vi "Get User Palette Choice.vi"(8 "Error In":errorcluster, 9 "Inverse (F)":bool, 10 "Interpolated Color Scale Definition":T1, 11 "Palette":string) -> (0 "Error Out":errorcluster, 1 "Palette Colors":u32[](array[numeric]), 2 "Palette Type":T2 items=["Grayscale", "Binary", "Gradient", "Rainbow", "Temperature", "User Defined", "Binary 16 Bit", "Gradient 16 Bit", "Rainbow 16 Bit", "Temperature 16 Bit", "User Defined 16 Bit"], 3 "Palette Name (# Colors)":string, 4 "Palette set?":bool, 5 "Brewer Palette?":bool, 6 "Interpolate?":bool)   [LabVIEW 2021]
uses:
  Image/Image Display Palette Type.ctl
  Interpolated Color Scale Definition.ctl
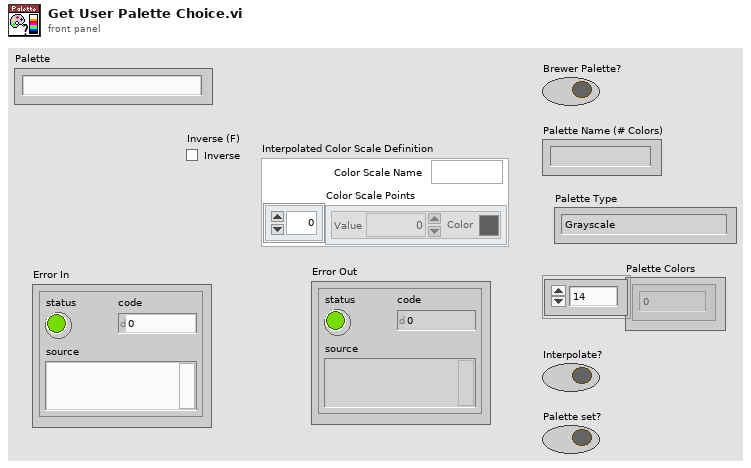
[diagram p1: front panel]
types:
  T1 = typedef "Interpolated Color Scale Definition.ctl" = cluster{"Color Scale Points":cluster{"Value":dbl, "Color":u32}[], "Color Scale Name":string}
  T2 = typedef "Image Display Palette Type.ctl" = u32
  T3 = typedef "Color Brewer Palette.ctl" = cluster{"Color Array":u32[], "Palette Name":string, "Number of Colors":i32, "Palette Category":string, "Color Blind Safe":bool, "Printer Friendly":bool, "Photocopy Safe":bool}
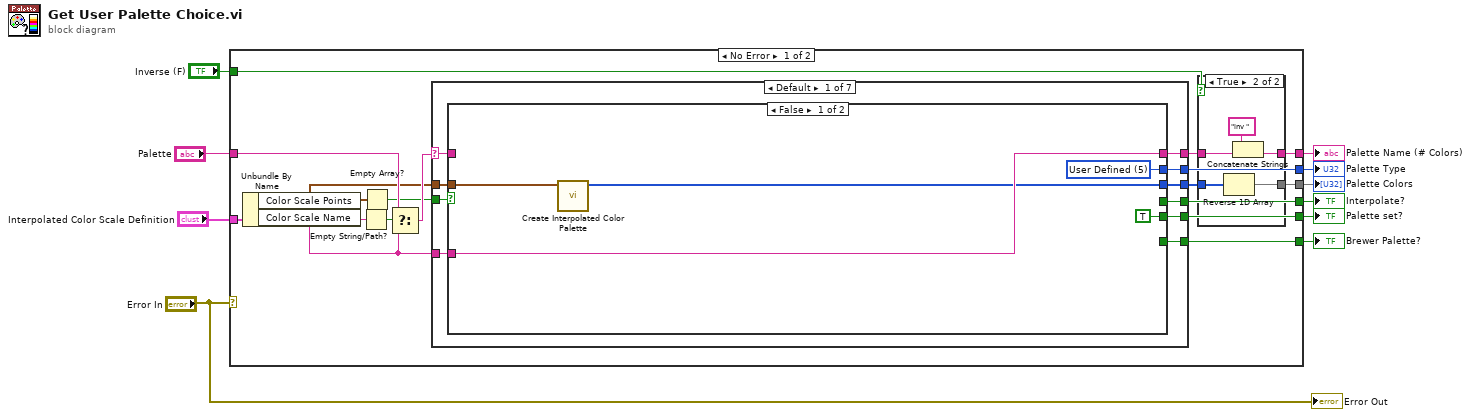
[diagram p0: block diagram]
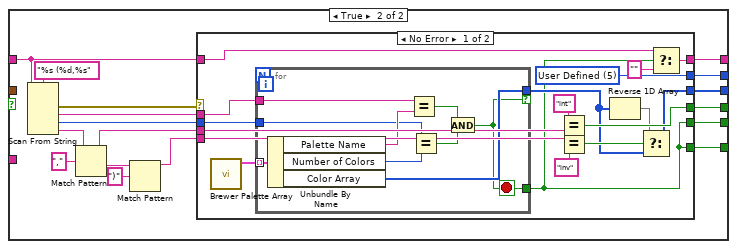
[diagram p3: hidden frame]
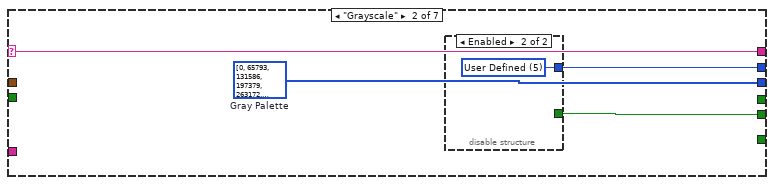
[diagram p5: hidden frame]
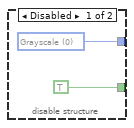
[diagram p6: hidden frame]
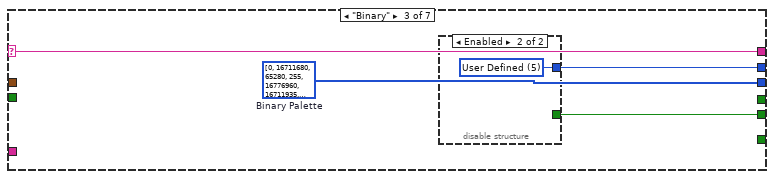
[diagram p7: hidden frame]
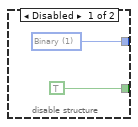
[diagram p8: hidden frame]
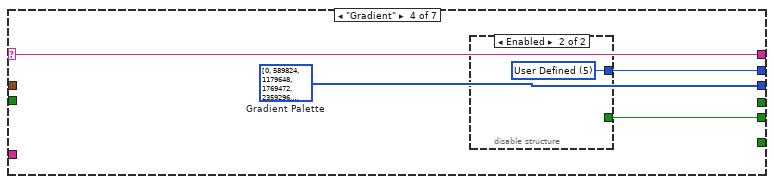
[diagram p9: hidden frame]
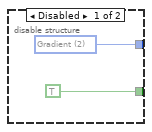
[diagram p10: hidden frame]
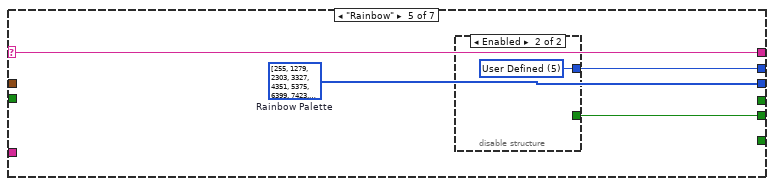
[diagram p11: hidden frame]
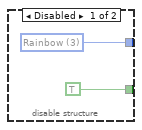
[diagram p12: hidden frame]
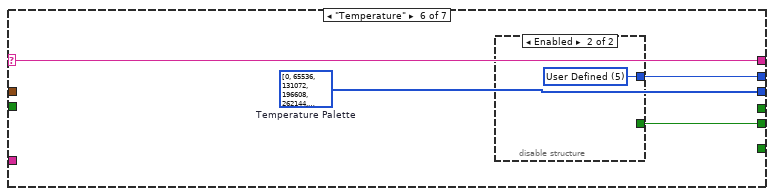
[diagram p13: hidden frame]
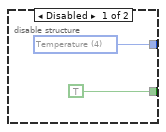
[diagram p14: hidden frame]
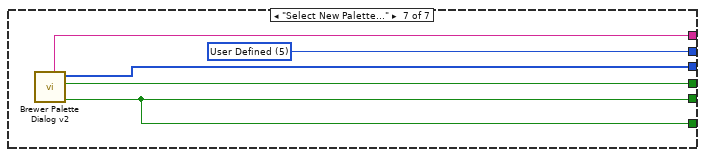
[diagram p15: hidden frame]
diagram:
  n1 = case shown="No Error" "Error In" {
    tunnel: [w20 _] -> w10
    tunnel: [w26 _] -> w9
    tunnel: [w18 _] -> w8
    tunnel: [w25 _] -> w7
    tunnel: [w24 _] -> w6
    tunnel: [w23 _] -> w5
    tunnel: "Palette" -> [w14 _]
    tunnel: "Inverse (F)" -> [w22 _]
    tunnel: "Interpolated Color Scale Definition" -> [w17 _]
    frame No Error {
      n2 = Unbundle By Name(w17) -> ("Color Scale Points"=w11:cluster{"Value":dbl, "Color":u32}[], "Color Scale Name"=w12:string)
      n3 = Empty String/Path?(string/path=w12) -> (empty?=w16:bool)
      n4 = Empty Array?(array=w11) -> (empty?=w13:bool)
      n5 = Select(t=w14, s=w16, f=w12) -> (s? t:f=w15:string)
      n6 = case shown="Default" w15 {
        selector: w15 -> [w37 w94 w101 w108 w115 w122 _]
        tunnel: [w41 w92 w99 w106 w113 w120 w131] -> w23
        tunnel: [w39 w95 w102 w109 w116 w123 w130] -> w24
        tunnel: [w42 _ _ _ _ _ w130] -> w25
        tunnel: [w43 w93 w100 w107 w114 w121 w129] -> w19
        tunnel: [w38 _ _ _ _ _ w128] -> w26
        tunnel: [w40 w94 w101 w108 w115 w122 w127] -> w21
        tunnel: w13 -> [w36 _ _ _ _ _ _]
        tunnel: w12 -> [w35 _ _ _ _ _ _]
        tunnel: w11 -> [w34 _ _ _ _ _ _]
        frame Default {
          n7 = case shown="False" w36 {
            tunnel: [w45 w62] -> w43
            tunnel: [_ w61] -> w42
            tunnel: [w47 w60] -> w41
            tunnel: [w48 w59] -> w40
            tunnel: [TRUE w58] -> w39
            tunnel: [_ w57] -> w38
            tunnel: w37 -> [_ w54]
            tunnel: w35 -> [w48 _]
            tunnel: w34 -> [w46 _]
            frame False {
              w47 = T2 5 items=["Grayscale", "Binary", "Gradient", "Rainbow", "Temperature", "User Defined", "Binary 16 Bit", "Gradient 16 Bit", "Rainbow 16 Bit", "Temperature 16 Bit", "User Defined 16 Bit"] ("Palette:Palette Type")
              n8 = call "Create Interpolated Color Palette.vi"("Color Scale Points"=w46) -> ("Interpolated Color Scale"=w45:u32[])  [unwired: 9 in, 1 out]
            }
            frame True {
              n9 = Scan From String(format string="%s (%d,%s", input string=w54) -> (error out=w65:errorcluster, output 1=w63:string, output 2=w64:i32, output 3=w52:string)  [unwired: 5 in, 2 out]
              n10 = Match Pattern(string=w52, regular expression=",") -> (before substring=w56:string, after substring=w50:string)  [unwired: 1 in, 2 out]
              n11 = Match Pattern(string=w50, regular expression=")") -> (before substring=w55:string)  [unwired: 1 in, 3 out]
              n12 = case shown="No Error" w65 {
                tunnel: w64 -> [w80 _]
                tunnel: w63 -> [w81 _]
                tunnel: [w70 _] -> w62
                tunnel: [w68 _] -> w61
                tunnel: [w79 _] -> w60
                tunnel: [w66 _] -> w59
                tunnel: [w68 _] -> w58
                tunnel: w56 -> [w78 _]
                tunnel: w55 -> [w75 _]
                tunnel: [w76 _] -> w57
                tunnel: w54 -> [w69 _]
                frame No Error {
                  w79 = T2 5 items=["Grayscale", "Binary", "Gradient", "Rainbow", "Temperature", "User Defined", "Binary 16 Bit", "Gradient 16 Bit", "Rainbow 16 Bit", "Temperature 16 Bit", "User Defined 16 Bit"] ("Palette:Palette Type")
                  n13 = call "Brewer Palette Array.vi"() -> ("Color Brewer Palette Array"=w82:T3[])  [unwired: 9 in]
                  n14 = for {
                    tunnel: w82 -> [w91] mode=indexing
                    tunnel: w81 -> [w84]
                    tunnel: w80 -> [w88]
                    tunnel: [w85] -> w72 if=w83
                    tunnel: [w83] -> w68
                    stop <- w83 stop-if-true
                    n15 = Unbundle By Name(w91) -> ("Palette Name"=w90:string, "Number of Colors"=w89:i32, "Color Array"=w85:u32[])
                    n16 = Equal?(x=w84, y=w90) -> (x = y?=w87:bool)
                    n17 = Equal?(x=w88, y=w89) -> (x = y?=w86:bool)
                    n18 = And(x=w87, y=w86) -> (x .and. y?=w83:bool)
                  }
                  n19 = Equal?(x="int", y=w78) -> (x = y?=w76:bool)
                  n20 = Equal?(x=w75, y="inv" ("x")) -> (x = y?=w73:bool)
                  n21 = Reverse 1D Array(array=w72) -> (reversed array=w71:u32[])
                  n22 = Select(t=w71, s=w73, f=w72) -> (s? t:f=w70:u32[])
                  n23 = Select(t=w69, s=w68, f="") -> (s? t:f=w66:string)
                }
                frame Error {
                }
              }
            }
          }
        }
        frame "Grayscale" {
          w93 = u32[] [0, 65793, 131586, 197379, 263172, 328965, 394758, 460551, 526344, 592137, 657930, 723723, 789516, 855309, 921102, 986895, 1052688, 1118481, 1184274, 1250067, 1315860, 1381653, 1447446, 1513239, 1579032, 1644825, 1710618, 1776411, 1842204, 1907997, 1973790, 2039583, 2105376, 2171169, 2236962, 2302755, 2368548, 2434341, 2500134, 2565927, 2631720, 2697513, 2763306, 2829099, 2894892, 2960685, 3026478, 3092271, 3158064, 3223857, 3289650, 3355443, 3421236, 3487029, 3552822, 3618615, 3684408, 3750201, 3815994, 3881787, 3947580, 4013373, 4079166, 4144959, 4210752, 4276545, 4342338, 4408131, 4473924, 4539717, 4605510, 4671303, 4737096, 4802889, 4868682, 4934475, 5000268, 5066061, 5131854, 5197647, 5263440, 5329233, 5395026, 5460819, 5526612, 5592405, 5658198, 5723991, 5789784, 5855577, 5921370, 5987163, 6052956, 6118749, 6184542, 6250335, 6316128, 6381921, 6447714, 6513507, 6579300, 6645093, 6710886, 6776679, 6842472, 6908265, 6974058, 7039851, 7105644, 7171437, 7237230, 7303023, 7368816, 7434609, 7500402, 7566195, 7631988, 7697781, 7763574, 7829367, 7895160, 7960953, 8026746, 8092539, 8158332, 8224125, 8289918, 8355711, 8421504, 8487297, 8553090, 8618883, 8684676, 8750469, 8816262, 8882055, 8947848, 9013641, 9079434, 9145227, 9211020, 9276813, 9342606, 9408399, 9474192, 9539985, 9605778, 9671571, 9737364, 9803157, 9868950, 9934743, 10000536, 10066329, 10132122, 10197915, 10263708, 10329501, 10395294, 10461087, 10526880, 10592673, 10658466, 10724259, 10790052, 10855845, 10921638, 10987431, 11053224, 11119017, 11184810, 11250603, 11316396, 11382189, 11447982, 11513775, 11579568, 11645361, 11711154, 11776947, 11842740, 11908533, 11974326, 12040119, 12105912, 12171705, 12237498, 12303291, 12369084, 12434877, 12500670, 12566463, 12632256, 12698049, 12763842, 12829635, 12895428, 12961221, 13027014, 13092807, 13158600, 13224393, 13290186, 13355979, 13421772, 13487565, 13553358, 13619151, 13684944, 13750737, 13816530, 13882323, 13948116, 14013909, 14079702, 14145495, 14211288, 14277081, 14342874, 14408667, 14474460, 14540253, 14606046, 14671839, 14737632, 14803425, 14869218, 14935011, 15000804, 15066597, 15132390, 15198183, 15263976, 15329769, 15395562, 15461355, 15527148, 15592941, 15658734, 15724527, 15790320, 15856113, 15921906, 15987699, 16053492, 16119285, 16185078, 16250871, 16316664, 16382457, 16448250, 16514043, 16579836, 16645629, 16711422, 16777215]  # Gray Palette
          n24 = disable-structure shown="Enabled" {
            disable-tunnel: [TRUE _] -> w95
            disable-tunnel: [w96 w98] -> w92
            frame Disabled {
              w96 = T2 0 items=["Grayscale", "Binary", "Gradient", "Rainbow", "Temperature", "User Defined", "Binary 16 Bit", "Gradient 16 Bit", "Rainbow 16 Bit", "Temperature 16 Bit", "User Defined 16 Bit"] ("Palette:Palette Type")
            }
            frame Enabled {
              w98 = T2 5 items=["Grayscale", "Binary", "Gradient", "Rainbow", "Temperature", "User Defined", "Binary 16 Bit", "Gradient 16 Bit", "Rainbow 16 Bit", "Temperature 16 Bit", "User Defined 16 Bit"] ("Palette:Palette Type")
            }
          }
        }
        frame "Binary" {
          w100 = u32[] [0, 16711680, 65280, 255, 16776960, 16711935, 65535, 16744192, 16711807, 8388352, 8323327, 32767, 65407, 16744319, 8388479, 8355839, 16711680, 65280, 255, 16776960, 16711935, 65535, 16744192, 16711807, 8388352, 8323327, 32767, 65407, 16744319, 8388479, 8355839, 16711680, 65280, 255, 16776960, 16711935, 65535, 16744192, 16711807, 8388352, 8323327, 32767, 65407, 16744319, 8388479, 8355839, 16711680, 65280, 255, 16776960, 16711935, 65535, 16744192, 16711807, 8388352, 8323327, 32767, 65407, 16744319, 8388479, 8355839, 16711680, 65280, 255, 16776960, 16711935, 65535, 16744192, 16711807, 8388352, 8323327, 32767, 65407, 16744319, 8388479, 8355839, 16711680, 65280, 255, 16776960, 16711935, 65535, 16744192, 16711807, 8388352, 8323327, 32767, 65407, 16744319, 8388479, 8355839, 16711680, 65280, 255, 16776960, 16711935, 65535, 16744192, 16711807, 8388352, 8323327, 32767, 65407, 16744319, 8388479, 8355839, 16711680, 65280, 255, 16776960, 16711935, 65535, 16744192, 16711807, 8388352, 8323327, 32767, 65407, 16744319, 8388479, 8355839, 16711680, 65280, 255, 16776960, 16711935, 65535, 16744192, 16711807, 8388352, 8323327, 32767, 65407, 16744319, 8388479, 8355839, 16711680, 65280, 255, 16776960, 16711935, 65535, 16744192, 16711807, 8388352, 8323327, 32767, 65407, 16744319, 8388479, 8355839, 16711680, 65280, 255, 16776960, 16711935, 65535, 16744192, 16711807, 8388352, 8323327, 32767, 65407, 16744319, 8388479, 8355839, 16711680, 65280, 255, 16776960, 16711935, 65535, 16744192, 16711807, 8388352, 8323327, 32767, 65407, 16744319, 8388479, 8355839, 16711680, 65280, 255, 16776960, 16711935, 65535, 16744192, 16711807, 8388352, 8323327, 32767, 65407, 16744319, 8388479, 8355839, 16711680, 65280, 255, 16776960, 16711935, 65535, 16744192, 16711807, 8388352, 8323327, 32767, 65407, 16744319, 8388479, 8355839, 16711680, 65280, 255, 16776960, 16711935, 65535, 16744192, 16711807, 8388352, 8323327, 32767, 65407, 16744319, 8388479, 8355839, 16711680, 65280, 255, 16776960, 16711935, 65535, 16744192, 16711807, 8388352, 8323327, 32767, 65407, 16744319, 8388479, 8355839, 16711680, 65280, 255, 16776960, 16711935, 65535, 16744192, 16711807, 8388352, 8323327, 32767, 65407, 16744319, 8388479, 16777215]  # Binary Palette
          n25 = disable-structure shown="Enabled" {
            disable-tunnel: [TRUE _] -> w102
            disable-tunnel: [w103 w105] -> w99
            frame Disabled {
              w103 = T2 1 items=["Grayscale", "Binary", "Gradient", "Rainbow", "Temperature", "User Defined", "Binary 16 Bit", "Gradient 16 Bit", "Rainbow 16 Bit", "Temperature 16 Bit", "User Defined 16 Bit"] ("Palette:Palette Type")
            }
            frame Enabled {
              w105 = T2 5 items=["Grayscale", "Binary", "Gradient", "Rainbow", "Temperature", "User Defined", "Binary 16 Bit", "Gradient 16 Bit", "Rainbow 16 Bit", "Temperature 16 Bit", "User Defined 16 Bit"] ("Palette:Palette Type")
            }
          }
        }
        frame "Gradient" {
          w107 = u32[] [0, 589824, 1179648, 1769472, 2359296, 2949120, 3538944, 4128768, 4718592, 5308416, 5898240, 6488064, 7077888, 7667712, 8257536, 8847360, 9437184, 9699328, 9961472, 10223616, 10485760, 10747904, 11010048, 11272192, 11534336, 11796480, 12058624, 12320768, 12582912, 12845056, 13107200, 13369344, 13631488, 13762560, 13893632, 14024704, 14155776, 14286848, 14417920, 14548992, 14680064, 14811136, 14942208, 15073280, 15204352, 15335424, 15466496, 15597568, 15728640, 15730176, 15731712, 15733248, 15734784, 15736320, 15737856, 15739392, 15740928, 15742464, 15744000, 15745536, 15747072, 15748608, 15750144, 15751680, 15753216, 15754240, 15755264, 15756288, 15757312, 15758336, 15759360, 15760384, 15761408, 15762432, 15763456, 15764480, 15765504, 15766528, 15767552, 15768576, 15769600, 15704832, 15640064, 15575296, 15510528, 15445760, 15380992, 15316224, 15251456, 15186688, 15121920, 15057152, 14992384, 14927616, 14862848, 14798080, 14733312, 14471680, 14210048, 13948416, 13686784, 13425152, 13163520, 12901888, 12640256, 12378624, 12116992, 11855360, 11593728, 11332096, 11070464, 10808832, 10547200, 10416134, 10285068, 10154002, 10022936, 9891870, 9760804, 9629738, 9498672, 9367606, 9236540, 9105474, 8974408, 8843342, 8712276, 8581210, 8450144, 8384613, 8319082, 8253551, 8188020, 8122489, 8056958, 7991427, 7925896, 7860365, 7794834, 7729303, 7663772, 7598241, 7532710, 7467179, 7401648, 7335603, 7269558, 7203513, 7137468, 7071423, 7005378, 6939333, 6873288, 6807243, 6741198, 6675153, 6609108, 6543063, 6477018, 6410973, 6344928, 6410465, 6476002, 6541539, 6607076, 6672613, 6738150, 6803687, 6869224, 6934761, 7000298, 7065835, 7131372, 7196909, 7262446, 7327983, 7393520, 7459312, 7525104, 7590896, 7656688, 7722480, 7788272, 7854064, 7919856, 7985648, 8051440, 8117232, 8183024, 8248816, 8314608, 8380400, 8446192, 8577519, 8708846, 8840173, 8971500, 9102827, 9234154, 9365481, 9496808, 9628135, 9759462, 9890789, 10022116, 10153443, 10284770, 10416097, 10547424, 10678496, 10809568, 10940640, 11071712, 11202784, 11333856, 11464928, 11596000, 11727072, 11858144, 11989216, 12120288, 12251360, 12382432, 12513504, 12644576, 12775648, 12906720, 13037792, 13168864, 13299936, 13431008, 13562080, 13693152, 13824224, 13955296, 14086368, 14217440, 14348512, 14479584, 14610656, 14741728, 14807265, 14872802, 14938339, 15003876, 15069413, 15134950, 15200487, 15266024, 15331561, 15397098, 15462635, 15528172, 15593709, 15659246, 15724783]  # Gradient Palette
          n26 = disable-structure shown="Enabled" {
            disable-tunnel: [TRUE _] -> w109
            disable-tunnel: [w110 w112] -> w106
            frame Disabled {
              w110 = T2 2 items=["Grayscale", "Binary", "Gradient", "Rainbow", "Temperature", "User Defined", "Binary 16 Bit", "Gradient 16 Bit", "Rainbow 16 Bit", "Temperature 16 Bit", "User Defined 16 Bit"] ("Palette:Palette Type")
            }
            frame Enabled {
              w112 = T2 5 items=["Grayscale", "Binary", "Gradient", "Rainbow", "Temperature", "User Defined", "Binary 16 Bit", "Gradient 16 Bit", "Rainbow 16 Bit", "Temperature 16 Bit", "User Defined 16 Bit"] ("Palette:Palette Type")
            }
          }
        }
        frame "Rainbow" {
          w114 = u32[] [255, 1279, 2303, 3327, 4351, 5375, 6399, 7423, 8447, 9471, 10495, 11519, 12543, 13567, 14591, 15615, 16639, 17663, 18687, 19711, 20735, 21759, 22783, 23807, 24831, 25855, 26879, 27903, 28927, 29951, 30975, 31999, 33023, 34047, 35071, 36095, 37119, 38143, 39167, 40191, 41215, 42239, 43263, 44287, 45311, 46335, 47359, 48383, 49407, 50431, 51455, 52479, 53503, 54527, 55551, 56575, 57599, 58623, 59647, 60671, 61695, 62719, 63743, 64767, 65535, 65531, 65527, 65523, 65519, 65515, 65511, 65507, 65503, 65499, 65495, 65491, 65487, 65483, 65479, 65475, 65471, 65467, 65463, 65459, 65455, 65451, 65447, 65443, 65439, 65435, 65431, 65427, 65423, 65419, 65415, 65411, 65407, 65403, 65399, 65395, 65391, 65387, 65383, 65379, 65375, 65371, 65367, 65363, 65359, 65355, 65351, 65347, 65343, 65339, 65335, 65331, 65327, 65323, 65319, 65315, 65311, 65307, 65303, 65299, 65295, 65291, 65287, 65283, 65280, 327424, 589568, 851712, 1113856, 1376000, 1638144, 1900288, 2162432, 2424576, 2686720, 2948864, 3211008, 3473152, 3735296, 3997440, 4259584, 4521728, 4783872, 5046016, 5308160, 5570304, 5832448, 6094592, 6356736, 6618880, 6881024, 7143168, 7405312, 7667456, 7929600, 8191744, 8453888, 8716032, 8978176, 9240320, 9502464, 9764608, 10026752, 10288896, 10551040, 10813184, 11075328, 11337472, 11599616, 11861760, 12123904, 12386048, 12648192, 12910336, 13172480, 13434624, 13696768, 13958912, 14221056, 14483200, 14745344, 15007488, 15269632, 15531776, 15793920, 16056064, 16318208, 16580352, 16776960, 16775936, 16774912, 16773888, 16772864, 16771840, 16770816, 16769792, 16768768, 16767744, 16766720, 16765696, 16764672, 16763648, 16762624, 16761600, 16760576, 16759552, 16758528, 16757504, 16756480, 16755456, 16754432, 16753408, 16752384, 16751360, 16750336, 16749312, 16748288, 16747264, 16746240, 16745216, 16744192, 16743168, 16742144, 16741120, 16740096, 16739072, 16738048, 16737024, 16736000, 16734976, 16733952, 16732928, 16731904, 16730880, 16729856, 16728832, 16727808, 16726784, 16725760, 16724736, 16723712, 16722688, 16721664, 16720640, 16719616, 16718592, 16717568, 16716544, 16715520, 16714496, 16713472, 16712448]  # Rainbow Palette
          n27 = disable-structure shown="Enabled" {
            disable-tunnel: [TRUE _] -> w116
            disable-tunnel: [w117 w119] -> w113
            frame Disabled {
              w117 = T2 3 items=["Grayscale", "Binary", "Gradient", "Rainbow", "Temperature", "User Defined", "Binary 16 Bit", "Gradient 16 Bit", "Rainbow 16 Bit", "Temperature 16 Bit", "User Defined 16 Bit"] ("Palette:Palette Type")
            }
            frame Enabled {
              w119 = T2 5 items=["Grayscale", "Binary", "Gradient", "Rainbow", "Temperature", "User Defined", "Binary 16 Bit", "Gradient 16 Bit", "Rainbow 16 Bit", "Temperature 16 Bit", "User Defined 16 Bit"] ("Palette:Palette Type")
            }
          }
        }
        frame "Temperature" {
          w121 = u32[] [0, 65536, 131072, 196608, 262144, 327680, 393216, 458752, 524288, 589824, 655360, 720896, 786432, 851968, 917504, 983040, 1048576, 1114112, 1179648, 1245184, 1310720, 1376256, 1441792, 1507328, 1572864, 1638400, 1703936, 1769472, 1835008, 1900544, 1966080, 2031616, 2097152, 2162688, 2228224, 2293760, 2359296, 2424832, 2490368, 2555904, 2621440, 2686976, 2752512, 2818048, 2883584, 2949120, 3014656, 3080192, 3145728, 3211264, 3276800, 3342336, 3407872, 3473408, 3538944, 3604480, 3670016, 3735552, 3801088, 3866624, 3932160, 3997696, 4063232, 4128768, 4194304, 4259840, 4325376, 4390912, 4456448, 4521984, 4587520, 4653056, 4718592, 4784128, 4849664, 4915200, 4980736, 5046272, 5111808, 5177344, 5242880, 5308416, 5373952, 5439488, 5505024, 5570560, 5636096, 5701632, 5767168, 5832704, 5898240, 5963776, 6029312, 6094848, 6160384, 6225920, 6291456, 6356992, 6422528, 6488064, 6553600, 6619136, 6684672, 6750208, 6815744, 6881536, 6947584, 7013632, 7079424, 7145472, 7211520, 7277312, 7343360, 7409408, 7475200, 7541248, 7607296, 7673088, 7739136, 7805184, 7871232, 7937024, 8003072, 8069120, 8134912, 8200960, 8267008, 8332800, 8398848, 8464896, 8530688, 8596736, 8662784, 8728576, 8794624, 8860672, 8926720, 8992512, 9058560, 9124608, 9190400, 9256448, 9322496, 9388290, 9454340, 9520390, 9586185, 9652235, 9718285, 9784079, 9850130, 9916180, 9982230, 10048024, 10114075, 10180125, 10245919, 10311969, 10378020, 10443814, 10509864, 10575914, 10641709, 10707759, 10773809, 10839859, 10905654, 10971704, 11037754, 11103548, 11169599, 11235649, 11301443, 11367493, 11433544, 11499338, 11565388, 11631438, 11697233, 11763283, 11829333, 11895384, 11961178, 12027228, 12093278, 12159073, 12225123, 12291173, 12356967, 12423018, 12489068, 12554862, 12620912, 12686963, 12752757, 12818807, 12884857, 12950908, 13016702, 13082752, 13148802, 13214597, 13280647, 13346697, 13412491, 13478542, 13544592, 13610386, 13676436, 13742487, 13808537, 13874331, 13940381, 14006432, 14072226, 14138276, 14204326, 14270121, 14336171, 14402221, 14468016, 14534066, 14600116, 14665910, 14731961, 14798011, 14864061, 14929855, 14995906, 15061956, 15127750, 15193800, 15259851, 15325645, 15391695, 15457745, 15523540, 15589590, 15655640, 15721434, 15787485, 15853535, 15919585, 15985379, 16051430, 16117480, 16183274, 16249324, 16315375, 16381169, 16447219, 16513269, 16579064, 16645114, 16711164, 16777215]  # Temperature Palette
          n28 = disable-structure shown="Enabled" {
            disable-tunnel: [TRUE _] -> w123
            disable-tunnel: [w124 w126] -> w120
            frame Disabled {
              w124 = T2 4 items=["Grayscale", "Binary", "Gradient", "Rainbow", "Temperature", "User Defined", "Binary 16 Bit", "Gradient 16 Bit", "Rainbow 16 Bit", "Temperature 16 Bit", "User Defined 16 Bit"] ("Palette:Palette Type")
            }
            frame Enabled {
              w126 = T2 5 items=["Grayscale", "Binary", "Gradient", "Rainbow", "Temperature", "User Defined", "Binary 16 Bit", "Gradient 16 Bit", "Rainbow 16 Bit", "Temperature 16 Bit", "User Defined 16 Bit"] ("Palette:Palette Type")
            }
          }
        }
        frame "Select New Palette..." {
          w131 = T2 5 items=["Grayscale", "Binary", "Gradient", "Rainbow", "Temperature", "User Defined", "Binary 16 Bit", "Gradient 16 Bit", "Rainbow 16 Bit", "Temperature 16 Bit", "User Defined 16 Bit"] ("Palette:Palette Type")
          n29 = call "Brewer Palette Dialog v2.vi"() -> ("OK?"=w130:bool, "Interpolate?"=w128:bool, "Selected Palette Colors"=w129:u32[], "Palette Name (# Colors)"=w127:string)  [unwired: 7 in, 1 out]
        }
      }
      n30 = case shown="True" w22 {
        tunnel: w21 -> [w28 w33]
        tunnel: [w28 w32] -> w20
        tunnel: w19 -> [w27 w30]
        tunnel: [w27 w29] -> w18
        frame False {
        }
        frame True {
          n31 = Reverse 1D Array(array=w30) -> (reversed array=w29:u32[])
          n32 = Concatenate Strings("inv " ("string"), w33) -> (w32:string)
        }
      }
    }
    frame Error {
    }
  }
  "Palette Name (# Colors)" <- w10
  "Interpolate?" <- w9
  "Palette Colors" <- w8
  "Brewer Palette?" <- w7
  "Palette set?" <- w6
  "Palette Type" <- w5
  "Error Out" <- "Error In"
